vi "RS232_命令(刀數).vi"(8 "error in (no error)":errorcluster, 9 "program":enum16{"0000", "0002"}(ring), 10 "刀數":u16, 11 "回復訊息 3":string) -> (0 "error out":errorcluster, 3 "result string 3":string)   [LabVIEW 2015]
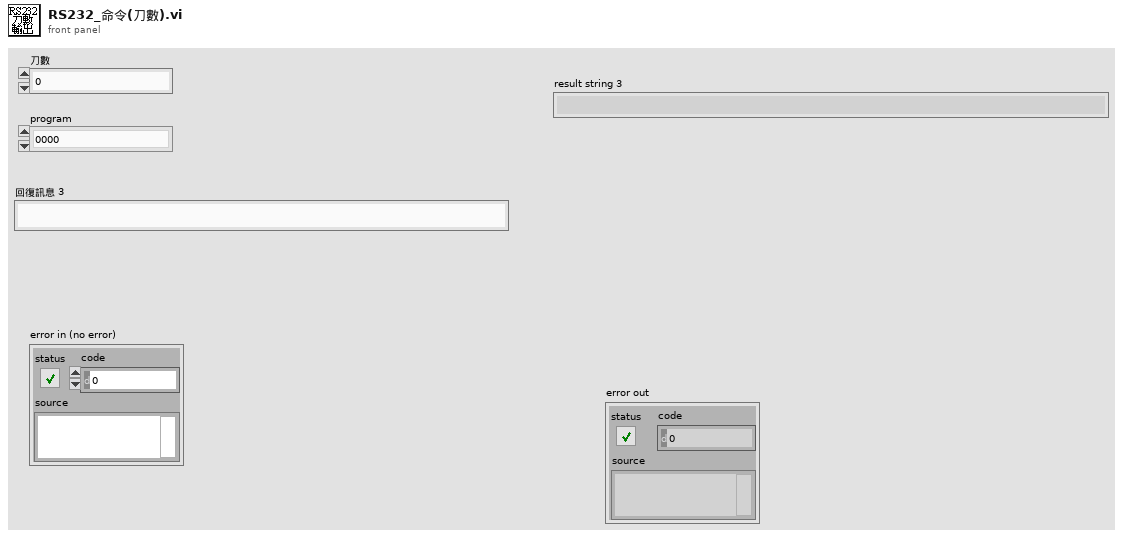
[diagram p1: front panel]
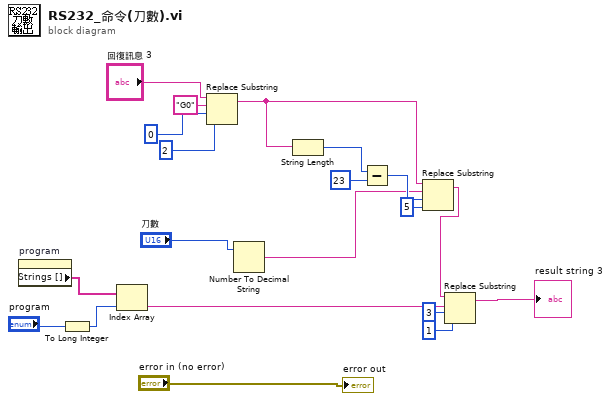
[diagram p0: block diagram]
diagram:
  n1 = property on="program" class="Enum (strict)"() -> ("Strings []"=w6:string[])  [unwired: 2 in, 2 out]
  n2 = To Long Integer(number="program") -> (32bit integer=w4:i32)
  n3 = Index Array(array=w6, index=w4) -> (element=w3:string)
  n4 = Replace Substring(2:2 ("length (len. of substring)"), 3:0 ("offset (0)"), 4:"G0" ("substring (\"\")"), 5:"回復訊息 3") -> (1:w12:string)  [unwired: 1 out]
  n5 = Number To Decimal String(number="刀數") -> (decimal integer string=w7:string)  [unwired: 1 in]
  n6 = String Length(string=w12) -> (length=w16:i32)
  n7 = Subtract(x=w16, y=23) -> (x-y=w14:i32)
  n8 = Replace Substring(2:5 ("length (len. of substring)"), 3:w14, 4:w7, 5:w12) -> (1:w1:string)  [unwired: 1 out]
  n9 = Replace Substring(2:1 ("length (len. of substring)"), 3:3 ("offset (0)"), 4:w3, 5:w1) -> (1:→"result string 3":string)  [unwired: 1 out]
  "error out" <- "error in (no error)"
